vi "ADDITION.vi"() -> ()   [LabVIEW 2010]
panel:
  out "c":u8
  in  "stop":bool
  in  "b":u8
  out "Waveform Chart":u8(graph)
  in  "A":u8
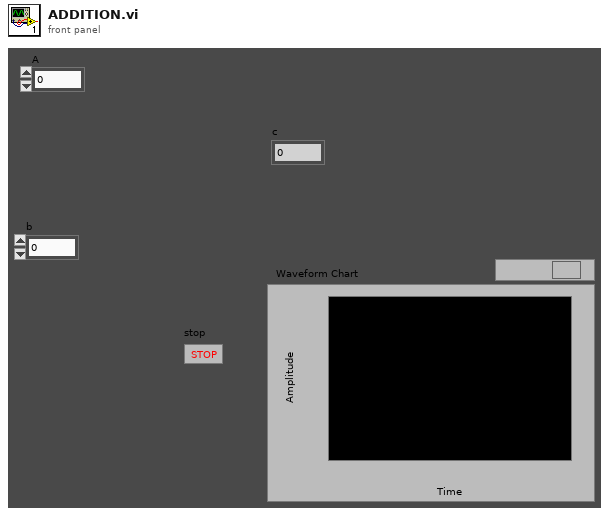
[diagram p1: front panel]
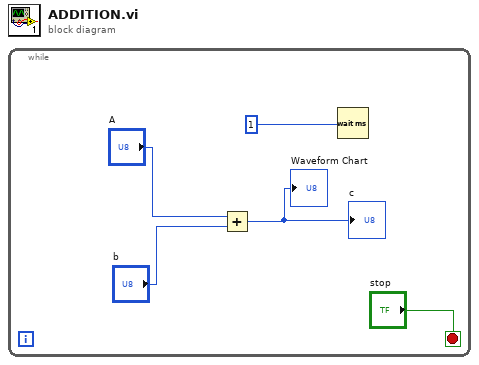
[diagram p0: block diagram]
diagram:
  n1 = while {
    stop <- "stop" stop-if-true
    n2 = Add(x="A", y="b") -> (x+y=→"c" →"Waveform Chart":u8)
    n3 = Wait (ms)(milliseconds to wait=u32 1 ("millisecond timer value")) -> ()  [unwired: 1 out]
  }
